vi "保存原始记录.vi"(8 "错误输入（无错误）":errorcluster, 11 "NI_report输入":refnum<class "NI_report.lvclass">) -> (0 "错误输出":errorcluster)   [LabVIEW 2015]
uses:
  <vilib>/Utility/NIReport.llb/NI_report.lvclass
  Global.vi
  <vilib>/addons/_office/excel.llb/Excel Get Data (str).vi
  <vilib>/addons/_office/NI_ReportGenerationToolkit.lvlib
  <vilib>/Utility/NIReport.llb/Excel/NI_Excel.lvclass
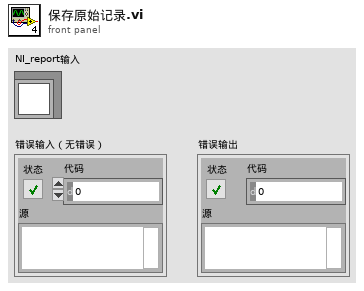
[diagram p1: front panel]
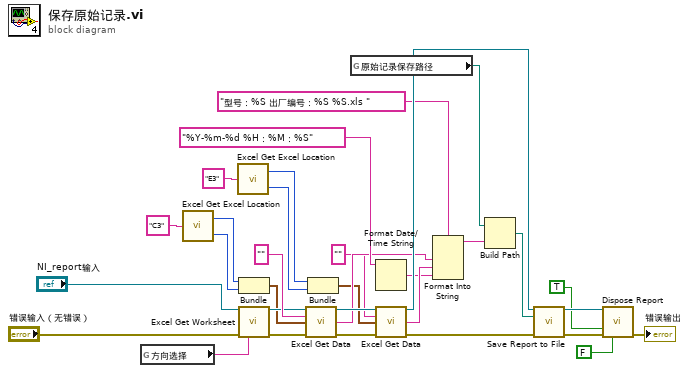
[diagram p0: block diagram]
diagram:
  n1 = global read "Global.vi" "方向选择"() -> (w1:string)
  n2 = call <vilib>:"Excel Get Excel Location.vi"("cell's name"="C3" ("data type")) -> ("row"=w8:i32, "column"=w7:i32)
  n3 = call <vilib>:"Excel Get Excel Location.vi"("cell's name"="E3" ("data type")) -> ("row"=w5:i32, "column"=w4:i32)
  n4 = Bundle("row"=w8, "column"=w7) -> (w6:cluster{"row":i32, "column":i32})  [unwired: 1 in]
  n5 = call <vilib>:"Excel Get Worksheet.vi"("report in"="NI_report输入", "error in (no error)"="错误输入（无错误）", "name (\"\")"=w1) -> ("report out"=w13:refnum<class "NI_report.lvclass">, "error out"=w12:errorcluster)  [unwired: 11 in]
  n6 = call-poly <vilib>:"Excel Get Data.vi"("report in"=w13, "data type"="", "start (0, 0)"=w6, "error in (no error)"=w12) -> ("report out"=w31:refnum<class "NI_report.lvclass">, "data"=w24:string, "error out"=w32:errorcluster)  [unwired: 9 in]
  n7 = Bundle("row"=w5, "column"=w4) -> (w3:cluster{"row":i32, "column":i32})  [unwired: 1 in]
  n8 = global read "Global.vi" "原始记录保存路径"() -> (w21:path)
  n9 = Format Date/Time String(time format string (%c)="%Y-%m-%d %H：%M：%S" ("时间格式字符串(%c)")) -> (date/time string=w22:string)  [unwired: 2 in]
  n10 = call-poly <vilib>:"Excel Get Data.vi"("report in"=w31, "data type"="", "start (0, 0)"=w3, "error in (no error)"=w32) -> ("report out"=w28:refnum<class "NI_report.lvclass">, "data"=w23:string, "error out"=w27:errorcluster)  [unwired: 9 in]
  n11 = Format Into String(format string="型号：%S 出厂编号：%S %S.xls " ("格式字符串"), w24, w23, w22) -> (resulting string=w20:string)  [unwired: 2 in, 1 out]
  n12 = Build Path(base path=w21, name or relative path=w20) -> (appended path=w19:path)
  n13 = call-dynamic "Save Report to File.vi"("report in"=w28, "report file path"=w19, "error in (no error)"=w27) -> ("report out"=w18:refnum<class "NI_report.lvclass">, "error out"=w17:errorcluster)  [unwired: 11 in]
  n14 = call-dynamic "Dispose Report.vi"("report in"=w18, "save changes? (F)"=TRUE, "error in (no error)"=w17, "close report? (T)"=FALSE ("save changes? (F)")) -> ("error out"=→"错误输出":errorcluster)  [unwired: 11 in]
